vi "DPT Config Read.vi"(0 "Config File Path":path=path "C:/work/flowconfig.ini", 11 "error in (no error)":errorcluster) -> (15 "error out":errorcluster)   [LabVIEW 2009]
uses:
  <vilib>/Utility/config.llb/Read Key (String).vi
  Dryer Performance/Global Test Variables DPT.vi
  <vilib>/Utility/config.llb/NI_LVConfig.lvlib
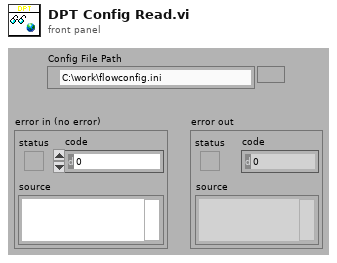
[diagram p1: front panel]
types:
  T1 = typedef "NI_LVConfig.lvlib/Config Data RefNum.ctl" = refnum<k1>
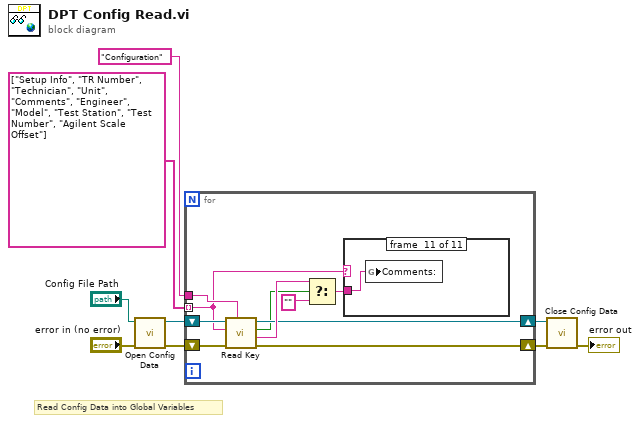
[diagram p0: block diagram]
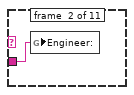
[diagram p3: hidden frame]
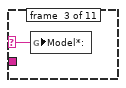
[diagram p4: hidden frame]
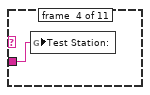
[diagram p5: hidden frame]
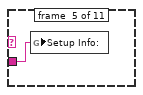
[diagram p6: hidden frame]
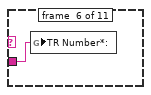
[diagram p7: hidden frame]
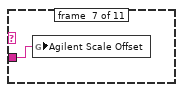
[diagram p8: hidden frame]
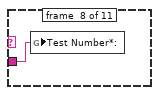
[diagram p9: hidden frame]
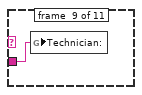
[diagram p10: hidden frame]
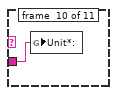
[diagram p11: hidden frame]
diagram:
  # "Read Config Data into Global Variables"
  n1 = call <vilib>:"Open Config Data.vi"("error in (no error)"="error in (no error)", "configuration file path"="Config File Path") -> ("error out"=w4:errorcluster, "refnum"=w5:T1)  [unwired: 7 in, 1 out]
  n2 = for {
    tunnel: "Configuration" ("key") -> [w17]
    tunnel: string[] ["Setup Info", "TR Number", "Technician", "Unit", "Comments", "Engineer", "Model", "Test Station", "Test Number", "Agilent Scale Offset"] -> [w16] mode=indexing
    shift-right: [w11] -> w6
    shift-left: w4 -> [w18]
    shift-right: [w12] -> w7
    shift-left: w5 -> [w19]
    n3 = call-poly <vilib>:"Read Key.vi"("section"=w17, "error in (no error)"=w18, "key"=w16, "refnum"=w19) -> ("error out"=w11:errorcluster, "value"=w15:string, "found?"=w10:bool, "refnum out"=w12:T1)  [unwired: 4 in]
    n4 = Select(t=w15, s=w10, f="") -> (s? t:f=w14:string)
    n5 = case shown="\"Agilent Scale Offset\"" w16 {
      selector: w16 -> [_ _ w21 _ _ _ _ _ _ _ _]
      tunnel: w14 -> [_ w20 _ w22 w23 w24 w25 w26 w27 w28 w29]
      frame #0 {
      }
      frame #1 {
        n6 = global write "Global Test Variables DPT.vi" "Engineer:"(w20) -> ()
      }
      frame #2 {
        n7 = global write "Global Test Variables DPT.vi" "Model*:"(w21) -> ()
      }
      frame #3 {
        n8 = global write "Global Test Variables DPT.vi" "Test Station:"(w22) -> ()
      }
      frame #4 {
        n9 = global write "Global Test Variables DPT.vi" "Setup Info:"(w23) -> ()
      }
      frame #5 {
        n10 = global write "Global Test Variables DPT.vi" "TR Number*:"(w24) -> ()
      }
      frame #6 {
        n11 = global write "Global Test Variables DPT.vi" "Agilent Scale Offset"(w25) -> ()
      }
      frame #7 {
        n12 = global write "Global Test Variables DPT.vi" "Test Number*:"(w26) -> ()
      }
      frame #8 {
        n13 = global write "Global Test Variables DPT.vi" "Technician:"(w27) -> ()
      }
      frame #9 {
        n14 = global write "Global Test Variables DPT.vi" "Unit*:"(w28) -> ()
      }
      frame #10 {
        n15 = global write "Global Test Variables DPT.vi" "Comments:"(w29) -> ()
      }
    }
  }
  n16 = call <vilib>:"Close Config Data.vi"("error in (no error)"=w6, "refnum"=w7) -> ("error out"=→"error out":errorcluster)  [unwired: 8 in, 1 out]
